vi "Build Timestamp.vi"(11 "record":T1 {"type" format="%04x"; "activity" format="%04x"; "error" format="%04x"; "cwd1" format="%04x"; "cwd2" format="%04x"; "swd1" format="%04x"; "swd2" format="%04x"; "data" format="%04x"}) -> (3 "timestamp":dbl)   [LabVIEW 2020, in "Ballard MIL-STD-1553 Engine.lvlib" / "Implementation.lvlib" / "Rx Execution Unit.lvclass"]
uses:
  Rx Execution Unit.lvclass
  <instrlib>/BTICardLib/Public/Controls/1553 Record.ctl
  <instrlib>/BTICardLib/BTICardLV.lvlib
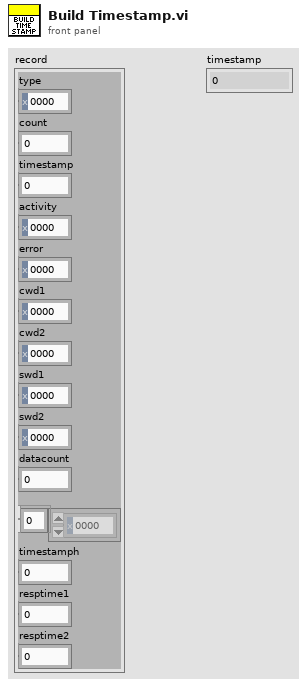
[diagram p1: front panel]
types:
  T1 = typedef "BTICardLV.lvlib/1553 Record.ctl" = cluster{"type":u16, "count":u16, "timestamp":u32, "activity":u16, "error":u16, "cwd1":u16, "cwd2":u16, "swd1":u16, "swd2":u16, "datacount":u16, "data":u16[], "timestamph":u32, "resptime1":u16, "resptime2":u16}
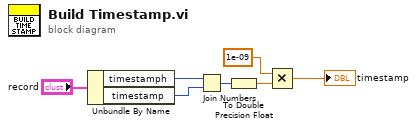
[diagram p0: block diagram]
diagram:
  n1 = Unbundle By Name("record") -> ("timestamph"=w3:u32, "timestamp"=w2:u32)
  n2 = Join Numbers(hi=w3, lo=w2) -> ((hi.lo)=w7:u64)
  n3 = To Double Precision Float(number=w7) -> (double precision float=w5:dbl)
  n4 = Multiply(x=1e-09 ("y"), y=w5) -> (x*y=→"timestamp":dbl)
